vi "NInstrSim_ConfigureWaveformFormat.appendData2Variant.vi"(0 "initData":variant, 2 "format (0:ASCII)":u16(ring) items=["ASCII", "8-bit Unsigned Binary", "16-bit Signed Binary"], 3 "byteOrder (0:Low Byte First)":u16(ring) items=["Low Byte First", "High Byte First"], 5 "error in (no error)":errorcluster) -> (14 "dup initData":variant, 19 "error out":errorcluster)   [LabVIEW 2009, in "HB_Device_Examples.lvlib" / "NInstrSim_ConfigureWaveformFormat.lvclass"]
doc: "Append initialize data to variant."
uses:
  NInstrSim_ConfigureWaveformFormat.lvclass
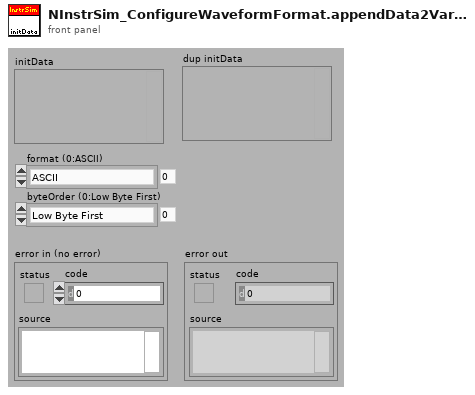
[diagram p1: front panel]
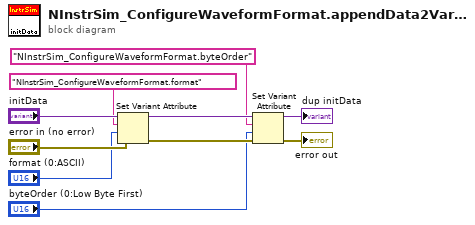
[diagram p0: block diagram]
diagram:
  n1 = Set Variant Attribute(Variant="initData", name="NInstrSim_ConfigureWaveformFormat.format", value="format (0:ASCII)", error in="error in (no error)") -> (Variant out=w5:variant, error out=w6:errorcluster)  [unwired: 1 out]
  n2 = Set Variant Attribute(Variant=w5, name="NInstrSim_ConfigureWaveformFormat.byteOrder", value="byteOrder (0:Low Byte First)", error in=w6) -> (Variant out=→"dup initData":variant, error out=→"error out":errorcluster)  [unwired: 1 out]
